vi "力特性计算.vi"(0 "左上升数组":dbl[][](array[numeric]), 1 "左下降数组":dbl[][](array[numeric]), 2 "测量点数组":dbl[](array[numeric]), 3 "右上升数组":dbl[][](array[numeric]), 4 "右下降数组":dbl[][](array[numeric])) -> (5 "对称度":dbl, 6 "左扭矩数组":dbl[](array[numeric]), 7 "右扭矩数组":dbl[](array[numeric]), 8 "扭差数组":dbl[](array[numeric]), 9 "左滞后数组":dbl[](array[numeric]), 10 "右滞后数组":dbl[](array[numeric]))   [LabVIEW 2013]
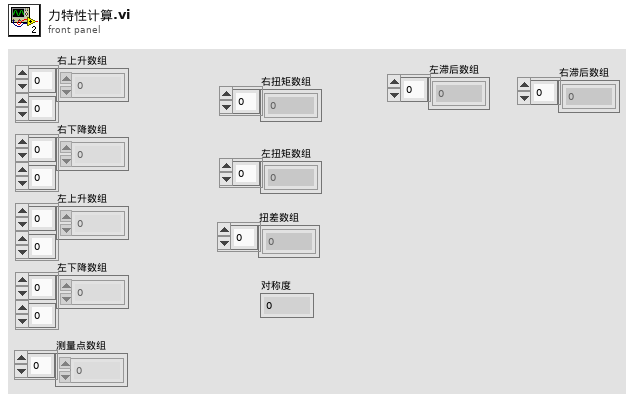
[diagram p1: front panel]
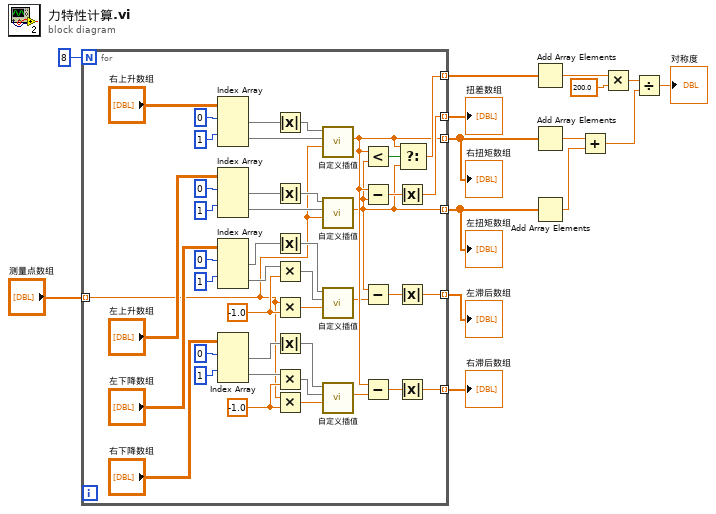
[diagram p0: block diagram]
diagram:
  n1 = for {
    N: 8 -> [_]
    tunnel: "测量点数组" -> [w18] mode=indexing
    tunnel: [w31] -> w3 mode=indexing
    tunnel: [w17] -> w4 mode=indexing
    tunnel: [w53] -> w5 mode=indexing
    tunnel: [w49] -> w6 mode=indexing
    tunnel: [w30] -> w2 mode=indexing
    tunnel: [w16] -> w1 mode=indexing
    w22 = -1.0 ("y")
    w40 = -1.0 ("y")
    n2 = Index Array(array="右上升数组", index (row) #1=0 ("索引 (行)"), index (row) #2=1 ("索引 (行)")) -> (element #1=w52:dbl[], element #2=w46:dbl[])  [unwired: 2 in]
    n3 = Index Array(array="左上升数组", index (row) #1=0 ("索引 (行)"), index (row) #2=1 ("索引 (行)")) -> (element #1=w51:dbl[], element #2=w44:dbl[])  [unwired: 2 in]
    n4 = Index Array(array="左下降数组", index (row) #1=0 ("索引 (行)"), index (row) #2=1 ("索引 (行)")) -> (element #1=w28:dbl[], element #2=w25:dbl[])  [unwired: 2 in]
    n5 = Index Array(array="右下降数组", index (row) #1=0 ("索引 (行)"), index (row) #2=1 ("索引 (行)")) -> (element #1=w33:dbl[], element #2=w37:dbl[])  [unwired: 2 in]
    n6 = Absolute Value(x=w52) -> (abs(x)=w45:dbl[])
    n7 = Absolute Value(x=w51) -> (abs(x)=w43:dbl[])
    n8 = Absolute Value(x=w28) -> (abs(x)=w27:dbl[])
    n9 = Multiply(x=w25, y=w22) -> (x*y=w24:dbl[])
    n10 = Multiply(x=w18, y=w22) -> (x*y=w23:dbl)
    n11 = Absolute Value(x=w33) -> (abs(x)=w34:dbl[])
    n12 = Multiply(x=w37, y=w40) -> (x*y=w38:dbl[])
    n13 = Multiply(x=w18, y=w40) -> (x*y=w39:dbl)
    n14 = call "自定义插值.vi"("压力"=w18, "压力数组"=w46, "扭矩数组"=w45) -> ("扭矩值"=w31:dbl)  [unwired: 8 in]
    n15 = call "自定义插值.vi"("压力"=w18, "压力数组"=w44, "扭矩数组"=w43) -> ("扭矩值"=w17:dbl)  [unwired: 8 in]
    n16 = call "自定义插值.vi"("压力"=w23, "压力数组"=w24, "扭矩数组"=w27) -> ("扭矩值"=w20:dbl)  [unwired: 8 in]
    n17 = call "自定义插值.vi"("压力"=w39, "压力数组"=w38, "扭矩数组"=w34) -> ("扭矩值"=w42:dbl)  [unwired: 8 in]
    n18 = Less?(x=w31, y=w17) -> (x < y?=w50:bool)
    n19 = Subtract(x=w31, y=w17) -> (x-y=w54:dbl)
    n20 = Subtract(x=w17, y=w20) -> (x-y=w21:dbl)
    n21 = Subtract(x=w31, y=w42) -> (x-y=w41:dbl)
    n22 = Absolute Value(x=w54) -> (abs(x)=w53:dbl)
    n23 = Absolute Value(x=w21) -> (abs(x)=w16:dbl)
    n24 = Absolute Value(x=w41) -> (abs(x)=w30:dbl)
    n25 = Select(t=w31, s=w50, f=w17) -> (s? t:f=w49:dbl)
  }
  "右扭矩数组" <- w3
  "左扭矩数组" <- w4
  "扭差数组" <- w5
  "右滞后数组" <- w2
  "左滞后数组" <- w1
  n26 = Add Array Elements(numeric array=w6) -> (sum=w11:dbl)
  n27 = Add Array Elements(numeric array=w3) -> (sum=w13:dbl)
  n28 = Add Array Elements(numeric array=w4) -> (sum=w12:dbl)
  n29 = Add(x=w13, y=w12) -> (x+y=w8:dbl)
  n30 = Multiply(x=w11, y=200.0) -> (x*y=w9:dbl)
  n31 = Divide(x=w9, y=w8) -> (x/y=→"对称度":dbl)
